vi "check_done.vi"(8 "error in (no error)":errorcluster, 11 "Waypoint in":refnum<class "Waypoint.lvclass">) -> (0 "error out":errorcluster, 2 "Done?":bool, 3 "Waypoint out":refnum<class "Waypoint.lvclass">)   [LabVIEW 2011, in "Waypoint.lvclass"]
uses:
  Waypoint.lvclass
  Waypoint.lvclass/Waypoint.ctl
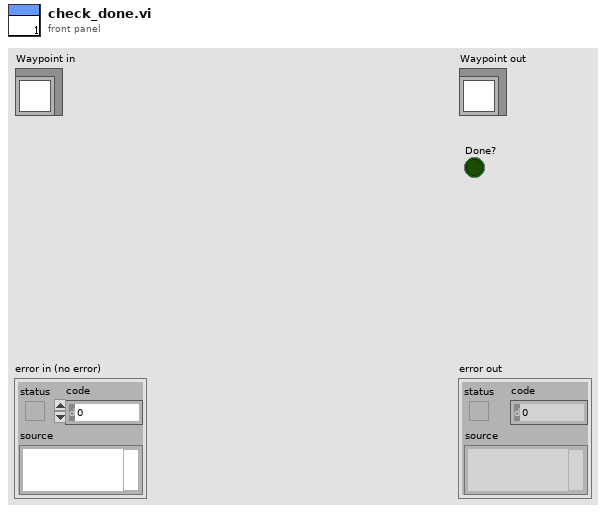
[diagram p1: front panel]
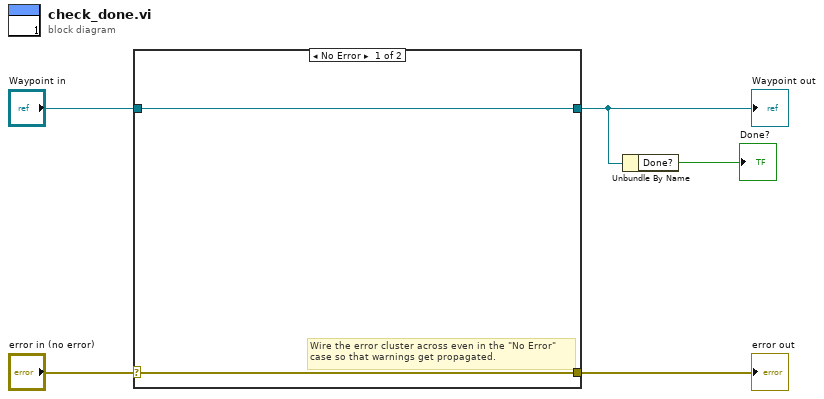
[diagram p0: block diagram]
diagram:
  n1 = case shown="No Error" "error in (no error)" {
    selector: "error in (no error)" -> [w6 w9]
    tunnel: [w6 w9] -> w4
    tunnel: [w7 w8] -> w2
    tunnel: "Waypoint in" -> [w7 w8]
    frame No Error {
      # "Wire the error cluster across even in the \"No Error\"\ncase so that warnings get propagated."
    }
    frame Error {
    }
  }
  "error out" <- w4
  "Waypoint out" <- w2
  n2 = Unbundle By Name(w2) -> ("Done?"=→"Done?":bool)
